vi "New.vi"(8 "error in (no error)":errorcluster, 9 "Group Type":T1, 10 "Parent":refnum<class "Config Element.lvclass">, 11 "Name":string) -> (0 "error out":errorcluster, 3 "Group out":refnum<class "Group.lvclass">)   [LabVIEW 2020, in "VolatusConfig.lvlib" / "Group.lvclass"]
uses:
  Group.lvclass
  C:/dev/lv20CE/relink/lv-volatus/VolatusConfig/VolatusConfigElement/VolatusConfigElement.lvclass
  lv-cdm/CDM-Config/Config Element/Config Element.lvclass
  Group Type.ctl
  Meta Type.ctl
  Meta Name.ctl
  lv-cdm/CDM-Config/Value Type.ctl
  Group.lvclass/Group.ctl
  lv-cdm/CDM-Config/CDM-Config.lvlib
  VolatusConfig.lvlib
  VolatusConfigElement/VolatusConfigElement.lvclass
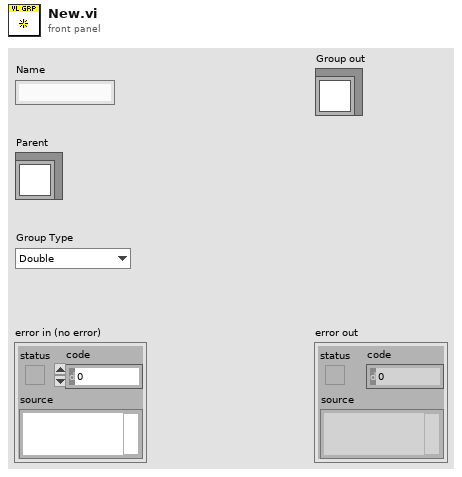
[diagram p1: front panel]
types:
  T1 = typedef "VolatusConfig.lvlib/Group Type.ctl" = enum16{"Double", "String"}
  T2 = typedef "CDM-Config.lvlib/Value Type.ctl" = enum16{"String", "Number", "Bool", "Object", "Array"}
  T3 = typedef "VolatusConfig.lvlib/Meta Name.ctl" = enum16{"VL_Type", "VL_Node_IP", "VL_Node_Type", "VL_Task_Type", "VL_Group_Type", "VL_Channel_Type", "VL_Channel_DataType", "VL_Config_Version", "VL_Overlay_Type"}
  T4 = typedef "VolatusConfig.lvlib/Meta Type.ctl" = enum16{"UNKNOWN", "VL_System", "VL_Cluster", "VL_Node", "VL_Task", "VL_Group", "VL_Channel", "VL_Task_List", "VL_Scaling", "VL_Sensor", "VL_Sensor_List", "VL_Scale"}
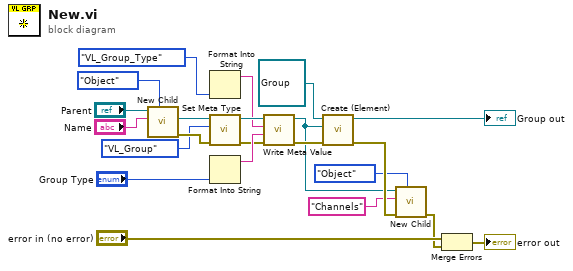
[diagram p0: block diagram]
diagram:
  n1 = call "New Child.vi"("Value Type (Object)"=Value_Type."Object" ("Value Type (String)"), "Child Name"="Name", "Config Element in"="Parent") -> ("error out"=w16:errorcluster, "New Child"=w17:refnum<class "Config Element.lvclass">)  [unwired: 6 in, 1 out]
  n2 = Format Into String(Meta_Name."VL_Group_Type" ("Meta Name")) -> (resulting string=w12:string)  [unwired: 3 in, 1 out]
  n3 = call "Set Meta Type.vi"("error in (no error)"=w16, "Meta Type"=Meta_Type."VL_Group", "Element In"=w17) -> ("error out"=w9:errorcluster, "Element"=w14:refnum<class "Config Element.lvclass">)  [unwired: 7 in]
  n4 = Format Into String("Group Type") -> (resulting string=w10:string)  [unwired: 3 in, 1 out]
  n5 = call "Write Meta Value.vi"("error in (no error)"=w9, "Meta Value"=w10, "Meta Name"=w12, "Config Element in"=w14) -> ("error out"=w7:errorcluster, "Config Element out"=w4:refnum<class "Config Element.lvclass">)  [unwired: 6 in]
  n6 = call "Create (Element).vi"("error in (no error)"=w7, "Element"=w4, "VolatusConfigElement in"=refnum<class "Group.lvclass"> refnum ("Group in")) -> ("error out"=w5:errorcluster, "VolatusConfigElement out"=→"Group out":refnum<class "Group.lvclass">)  [unwired: 7 in]
  n7 = call "New Child.vi"("Value Type (Object)"=Value_Type."Object" ("Value Type (String)"), "error in (no error)"=w5, "Child Name"="Channels", "Config Element in"=w4) -> ("error out"=w1:errorcluster)  [unwired: 5 in, 2 out]
  n8 = Merge Errors("error in (no error)", w1) -> (→"error out":errorcluster)
